vi "ATFileExistAddOne.vi"(10 "input string":string="2014/10/03") -> (2 "appended path":path)   [LabVIEW 2012]
uses:
  Global1.vi
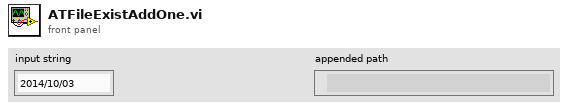
[diagram p1: front panel]
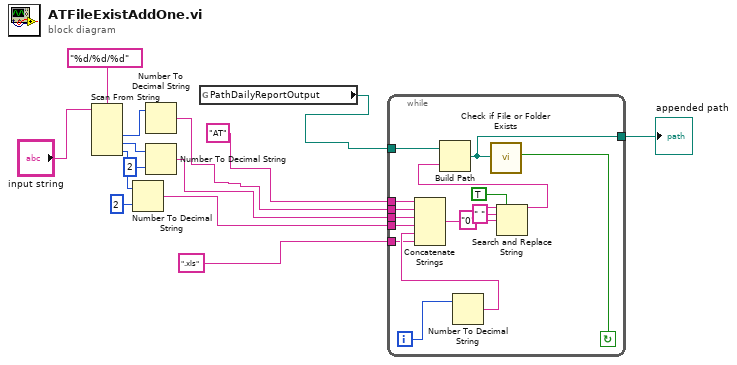
[diagram p0: block diagram]
diagram:
  n1 = Scan From String(format string="%d/%d/%d", input string="input string") -> (output 1=w13:i32, output 2=w12:i32, output 3=w11:i32)  [unwired: 5 in, 3 out]
  n2 = Number To Decimal String(number=w11, width (-)=i16 2) -> (decimal integer string=w2:string)
  n3 = Number To Decimal String(number=w13) -> (decimal integer string=w6:string)  [unwired: 1 in]
  n4 = Number To Decimal String(number=w12, width (-)=i16 2) -> (decimal integer string=w5:string)
  n5 = global read "Global1.vi" "PathDailyReportOutput"() -> (w9:path)
  n6 = while {
    tunnel: w9 -> [w29]
    tunnel: [w27] -> w8
    tunnel: "AT" ("string") -> [w25]
    tunnel: w6 -> [w24]
    tunnel: w5 -> [w23]
    tunnel: w2 -> [w22]
    tunnel: ".xls" ("string") -> [w20]
    i -> [w26]
    stop <- w28 continue-if-true
    n7 = Number To Decimal String(number=w26) -> (decimal integer string=w21:string)  [unwired: 1 in]
    n8 = Concatenate Strings(w25, w24, w23, w22, w21, w20) -> (w19:string)
    n9 = Search and Replace String(replace all?=TRUE ("replace all? (F)"), input string=w19, search string=" ", replace string="0" ("replace string (\"\")")) -> (result string=w15:string)  [unwired: 4 in, 3 out]
    n10 = Build Path(base path=w29, name or relative path=w15) -> (appended path=w27:path)
    n11 = call <vilib>:"Check if File or Folder Exists.vi"("path"=w27) -> ("file or folder exists?"=w28:bool)  [unwired: 8 in, 2 out]
  }
  "appended path" <- w8
